vi "Scaling Dead Zone.vi"(4 "Input":dbl) -> (1 "Output":dbl)   [LabVIEW 2015]
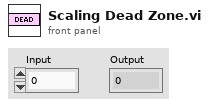
[diagram p1: front panel]
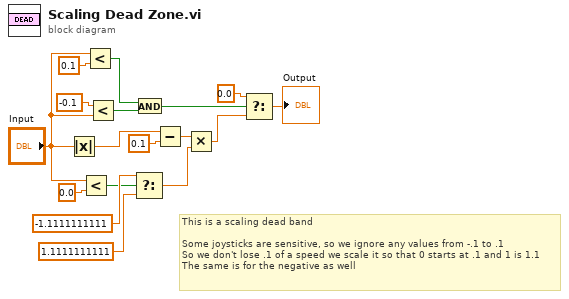
[diagram p0: block diagram]
diagram:
  # "This is a scaling dead band\n\nSome joysticks are sensitive, so we ignore any values from -.1 to .1\nSo we don't lose .1 of a speed we scale it so that 0 starts at .1 and 1 is 1.1\nThe same is for the negative as well"
  n1 = Absolute Value(x="Input") -> (abs(x)=w7:dbl)
  n2 = Less?(x="Input", y=0.0) -> (x < y?=w11:bool)
  n3 = Less?(x="Input", y=0.1) -> (x < y?=w4:bool)
  n4 = Less?(x=-0.1, y="Input") -> (x < y?=w3:bool)
  n5 = Select(t=-1.1111111111, s=w11, f=1.1111111111) -> (s? t:f=w12:dbl)
  n6 = And(x=w4, y=w3) -> (x .and. y?=w5:bool)
  n7 = Subtract(x=w7, y=0.1) -> (x-y=w10:dbl)
  n8 = Multiply(x=w10, y=w12) -> (x*y=w15:dbl)
  n9 = Select(t=0.0, s=w5, f=w15) -> (s? t:f=→"Output":dbl)
